vi "Configure Optimum Attenuator for Mixer IMD.vi"(7 "Use Eletronic Attenuator (F)":bool, 8 "error in (no error)":errorcluster, 9 "Frequency offset between F1 and F2":dbl, 10 "Power Level at SA":dbl, 11 "MXA in":refnum<class "MXA.lvclass">) -> (0 "error out":errorcluster, 3 "MXA out":refnum<class "MXA.lvclass">)   [LabVIEW 2020, in "MXA.lvclass"]
uses:
  MXA.lvclass
  C:/Sandbox/RF Bench/Source Code/WiSpry Test Framework/Instruments/Spectrum Analyzer/Spectrum Analyzer.lvclass
  Spectrum Analyzer.lvclass/Spectrum Analyzer.ctl
  Spectrum Analyzer.lvclass
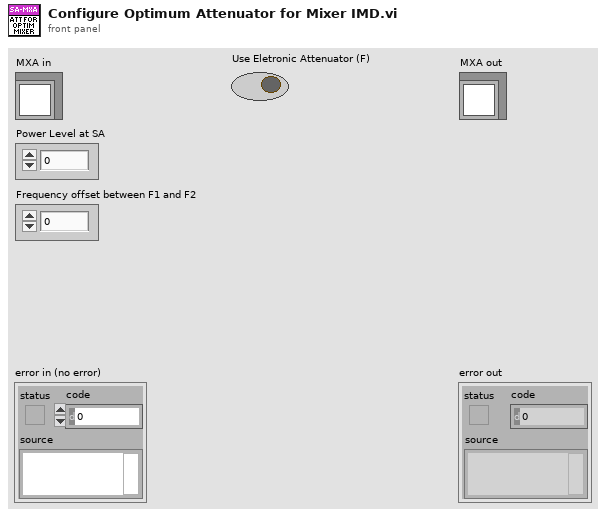
[diagram p1: front panel]
types:
  T1 = cluster{"Offset Frequency":dbl, "Mixer Level":dbl}[]
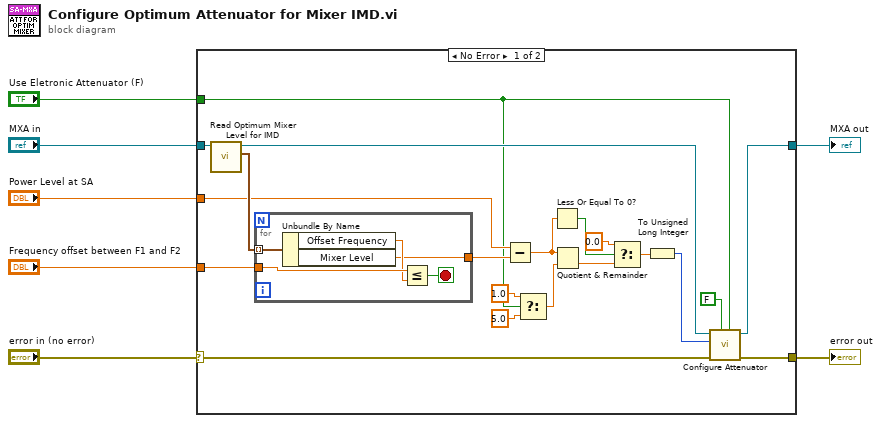
[diagram p0: block diagram]
diagram:
  n1 = case shown="No Error" "error in (no error)" {
    selector: "error in (no error)" -> [w9 w34]
    tunnel: "MXA in" -> [w25 w33]
    tunnel: [w10 w34] -> w6
    tunnel: [w11 w33] -> w5
    tunnel: "Frequency offset between F1 and F2" -> [w26 _]
    tunnel: "Power Level at SA" -> [w14 _]
    tunnel: "Use Eletronic Attenuator (F)" -> [w8 _]
    frame No Error {
      n2 = call "Read Optimum Mixer Level for IMD.vi"("Spectrum Analyzer in"=w25) -> ("Optimum Mixer Level for IMD"=w27:T1, "Spectrum Analyzer out"=w24:refnum<class "MXA.lvclass">)  [unwired: 9 in]
      n3 = for {
        tunnel: w27 -> [w32] mode=indexing
        tunnel: w26 -> [w31]
        tunnel: [w28] -> w15
        stop <- w29 stop-if-true
        n4 = Unbundle By Name(w32) -> ("Offset Frequency"=w30:dbl, "Mixer Level"=w28:dbl)
        n5 = Less Or Equal?(x=w31, y=w30) -> (x <= y?=w29:bool)
      }
      n6 = Subtract(x=w14, y=w15) -> (x-y=w18:dbl)
      n7 = Select(t=1.0, s=w8, f=5.0) -> (s? t:f=w19:dbl)
      n8 = Less Or Equal To 0?(x=w18) -> (x <= 0?=w23:bool)
      n9 = Quotient & Remainder(x=w18, y=w19) -> (floor(x/y)=w17:dbl)  [unwired: 1 out]
      n10 = Select(t=0.0, s=w23, f=w17) -> (s? t:f=w16:dbl)
      n11 = To Unsigned Long Integer(number=w16) -> (unsigned 32bit integer=w12:u32)
      n12 = call-dynamic "Configure Attenuator.vi"("Use Eletronic Attenuator (F)"=w8, "Auto Attenuator (T)"=FALSE, "error in (no error)"=w9, "Attenuator (dB)"=w12, "MXA in"=w24) -> ("error out"=w10:errorcluster, "MXA out"=w11:refnum<class "MXA.lvclass">)  [unwired: 5 in]
    }
    frame Error {
    }
  }
  "error out" <- w6
  "MXA out" <- w5
